vi "PythonCodes.vi"() -> ()   [LabVIEW 2022 SP3]
uses:
  <vilib>/event_ctls.llb/eventvkey.ctl
panel:
  out "VKey":T1
  in  "stop":bool
  in  "Python Code":string
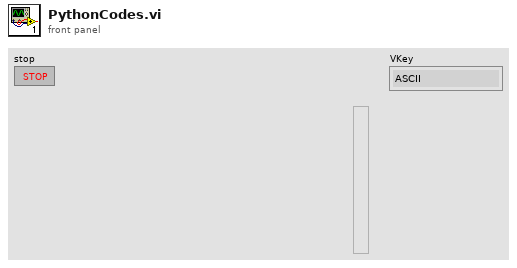
[diagram p1: front panel]
types:
  T1 = typedef "eventvkey.ctl" = enum16{"ASCII", "Enter", "Return", "Shift", "Ctrl", "Alt", "Cmd", "Opt", "Caps", "NumLock", "Clear", "Break", "Up", "Down", "Left", "Right", "Insert", "Delete", "Home", "End", "PageUp", "PageDown", "Escape", "Help", "Pause", "ScrollLock", "F1", "F2", "F3", "F4", "F5", "F6", "F7", "F8", "F9", "F10", "F11", "F12", "F13", "F14", "F15", "F16", "F17", "F18", "F19", "F20", "F21", "F22", "F23", "F24", "Play", "VolumeUp", "VolumeDown", "Mute", "Two Byte Char"}
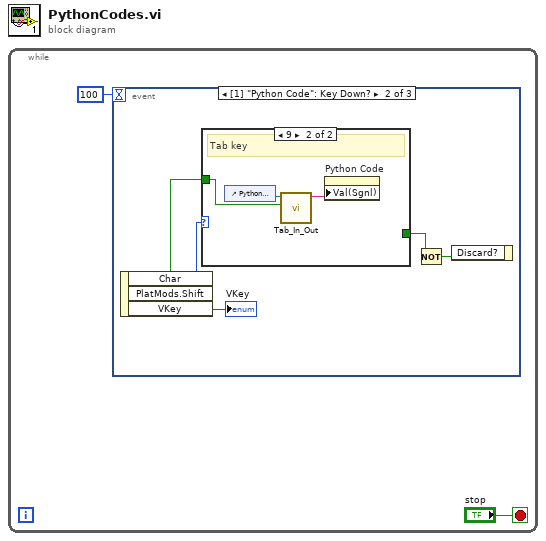
[diagram p0: block diagram]
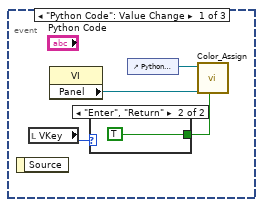
[diagram p2: hidden frame]
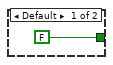
[diagram p3: hidden frame]
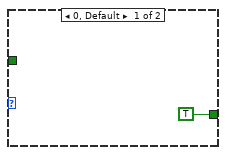
[diagram p4: hidden frame]
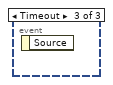
[diagram p5: hidden frame]
diagram:
  n1 = while {
    stop <- "stop" stop-if-true
    n2 = event shown="[1] \"Python Code\": Key Down?" {
      selector: _ -> [_ _ _]
      dyn-events: _ -> [_ _ _]
      timeout: 100 -> [_ _ _]
      event "Python Code": Value Change {
        n3 = event-data() -> ()  [unwired: 1 in, 1 out]
        n4 = local read "VKey"() -> (w3:T1)
        n5 = property class="VI"() -> ("Panel"=w5:refnum<vi>)  [unwired: 2 in, 2 out]
        n6 = case shown="\"Enter\", \"Return\"" w3 {
          tunnel: [FALSE TRUE] -> w4
          frame Default {
          }
          frame "Enter", "Return" {
          }
        }
        n7 = control-ref of="Python Code"() -> (w6:refnum<vi>)
        n8 = call "Color_Assign.vi"("Add Spaces?"=w4, "Front Panel"=w5, "Code"=w6) -> ()  [unwired: 8 in, 1 out]
      }
      event "Python Code": Key Down? {
        n9 = event-data() -> ("Char"=w9:i16, "PlatMods.Shift"=w10:bool, "VKey"=→"VKey":T1)  [unwired: 1 in]
        n10 = case shown="9" w9 {
          tunnel: [TRUE ("Discard?") _] -> w12
          tunnel: w10 -> [_ w16]
          frame 0, Default {
          }
          frame 9 {
            # "Tab key"
            n11 = control-ref of="Python Code"() -> (w17:refnum<vi>)
            n12 = call "Tab_In_Out.vi"("Shift?"=w16, "String in"=w17) -> ("result string"=w15:string)  [unwired: 9 in]
            n13 = property on="Python Code" class="Str"("Val(Sgnl)"=w15) -> ()  [unwired: 2 in, 2 out]
          }
        }
        n14 = Not(x=w12) -> (.not. x?=w11:bool)
        n15 = event-data("Discard?"=w11) -> ()  [unwired: 1 in, 1 out]
      }
      event Timeout {
        n16 = event-data() -> ()  [unwired: 1 in, 1 out]
      }
    }
  }
